vi "LoopClockLuncher.vi"(6 "Instance":i32, 7 "Loop VI Depth":i32=1, 8 "error in (no error)":errorcluster, 10 "milliseconds to wait":i32=200) -> (0 "error out":errorcluster, 3 "reference out":refnum<vi>)   [LabVIEW 2017, in "Communication.lvlib"]
uses:
  Communication.lvlib
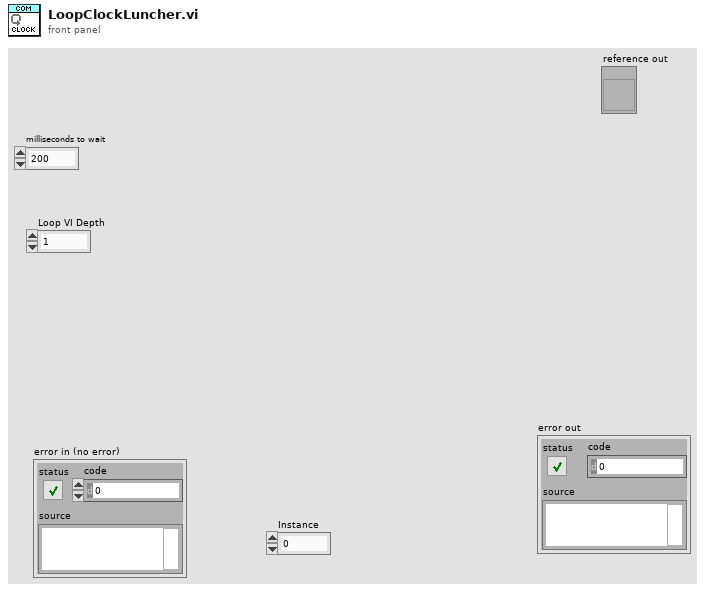
[diagram p1: front panel]
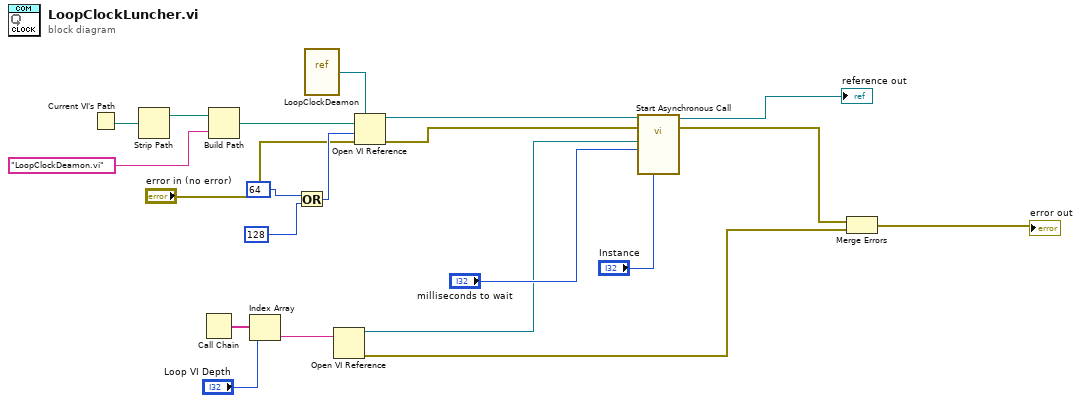
[diagram p0: block diagram]
diagram:
  n1 = Current VI's Path() -> (path=w20:path)
  n2 = Strip Path(path=w20) -> (stripped path=w19:path)  [unwired: 1 out]
  n3 = Call Chain() -> (call chain=w7:string[])
  n4 = Build Path(base path=w19, name or relative path="LoopClockDeamon.vi") -> (appended path=w17:path)
  n5 = Index Array(array=w7, index="Loop VI Depth") -> (element=w5:string)
  n6 = Or(x=64 ("options"), y=128 ("options")) -> (x .or. y?=w14:i32)
  n7 = vi-ref "LoopClockDeamon.vi"() -> (w21:refnum<vi>)
  n8 = Open VI Reference(vi path=w5) -> (vi reference=w1:refnum<vi>, error out=w2:errorcluster)  [unwired: 5 in]
  n9 = Open VI Reference(type specifier VI Refnum (for type only)=w21, vi path=w17, options=w14, error in (no error)="error in (no error)") -> (vi reference=w13:refnum<vi>, error out=w12:errorcluster)  [unwired: 2 in]
  n10 = call-by-ref "Start Asynchronous Call"(reference=w13, error in=w12, "Instance"="Instance", "milliseconds to wait"="milliseconds to wait", "VI Refnum"=w1) -> (reference out=→"reference out":refnum<vi>, error out=w4:errorcluster)  [unwired: 9 in]
  n11 = Merge Errors(w4, w2) -> (→"error out":errorcluster)
